vi "PV Curtail Hz.vi"(5 "1/I":dbl=1.0, 6 "PVCurtailEnable":bool, 7 "P":dbl=0.01, 8 "Error In":errorcluster, 9 "reinitialize? (F)":bool, 10 "Current Limit Output":T2, 11 "FPGA Data":T1 {"SSG Active Current" format="%2.1f"; "PV Reactive Power (L1)" format="%2.1f"; "PV Reactive Power (L2)" format="%2.1f"; "PV Total Reactive Power" format="%2.1f"; "Gen Reactive Power (L1)" format="%2.1f"; "Gen Reactive Power (L2)" format="%2.1f"; "Gen Total Reactive Power" format="%2.1f"; "SSG Reactive Power (L1)" format="%2.1f"; "SSG Reactive Power (L2)" format="%2.1f"; "SSG Total Reactive Power" format="%2.1f"; "PV Total Current" format="%2.1f"; "PV Total Voltage" format="%2.1f"; "PV Active Power (L1)" format="%2.1f"; "PV Active Power (L2)" format="%2.1f"; "PV App Power (L1)" format="%2.1f"; "PV App Power (L2)" format="%2.1f"; "PV Total Active Power" format="%2.1f"; "PV Total App Power" format="%2.1f"; "PV Arms (L1)" format="%2.1f"; "PV Arms (L2)" format="%2.1f"; "PV Vrms (L1)" format="%2.1f"; "PV Vrms (L2)" format="%2.1f"; "Gen Total Current" format="%2.1f"; "SSG Total Current" format="%2.1f"; "Gen Total Voltage" format="%2.1f"; "SSG Total Voltage" format="%2.1f"; "Gen Active Power (L1)" format="%2.1f"; "Gen Active Power (L2)" format="%2.1f"; "SSG Active Power (L1)" format="%2.1f"; "SSG Active Power (L2)" format="%2.1f"; "Gen App Power (L1)" format="%2.1f"; "Gen App Power (L2)" format="%2.1f"; "SSG App Power (L1)" format="%2.1f"; "SSG App Power (L2)" format="%2.1f"; "Gen Total Active Power" format="%2.1f"; "Gen Total App Power" format="%2.1f"; "Gen Arms (L1)" format="%2.1f"; "Gen Arms (L2)" format="%2.1f"; "Gen Vrms (L1)" format="%2.1f"; "Gen Vrms (L2)" format="%2.1f"; "SSG Total Active Power" format="%2.1f"; "SSG Total App Power" format="%2.1f"; "SSG Arms (L1)" format="%2.1f"; "SSG Arms (L2)" format="%2.1f"; "SSG Vrms (L1)" format="%2.1f"; "SSG Vrms (L2)" format="%2.1f"}) -> (0 "Error Out":errorcluster, 3 "Frequency Setpoint":sgl)   [LabVIEW 2014]
uses:
  Controls/Current Limit Output.ctl
  Controls/FPGA Data.ctl
  <vilib>/functionblocks/Control/PID/PID.vi
  <vilib>/functionblocks/FB Core/FB Core.xnode
  <vilib>/functionblocks/NI_FunctionBlock Libraries.lvlib
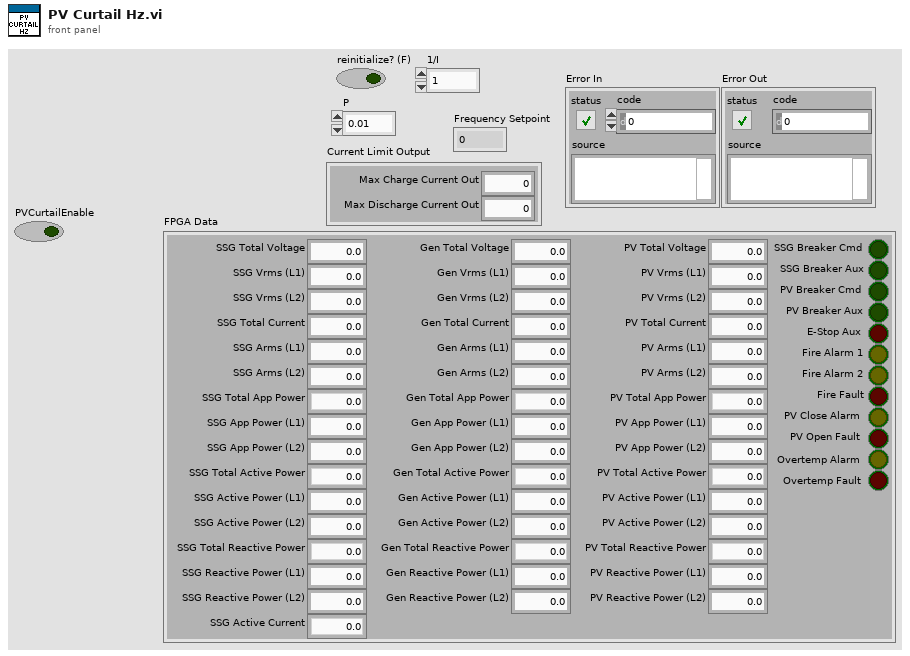
[diagram p1: front panel]
types:
  T1 = typedef "FPGA Data.ctl" = cluster{"Gen Total Voltage":dbl, "Gen Vrms (L1)":dbl, "Gen Vrms (L2)":dbl, "Gen Total Current":dbl, "Gen Arms (L1)":dbl, "Gen Arms (L2)":dbl, "Gen Total App Power":dbl, "Gen App Power (L1)":dbl, "Gen App Power (L2)":dbl, "Gen Total Active Power":dbl, "Gen Active Power (L1)":dbl, "Gen Active Power (L2)":dbl, "Gen Total Reactive Power":dbl, "Gen Reactive Power (L1)":dbl, "Gen Reactive Power (L2)":dbl, "SSG Total Voltage":dbl, "SSG Vrms (L1)":dbl, "SSG Vrms (L2)":dbl, "SSG Total Current":dbl, "SSG Arms (L1)":dbl, "SSG Arms (L2)":dbl, "SSG Total App Power":dbl, "SSG App Power (L1)":dbl, "SSG App Power (L2)":dbl, "SSG Total Active Power":dbl, "SSG Active Power (L1)":dbl, "SSG Active Power (L2)":dbl, "SSG Total Reactive Power":dbl, "SSG Reactive Power (L1)":dbl, "SSG Reactive Power (L2)":dbl, "PV Total Voltage":dbl, "PV Vrms (L1)":dbl, "PV Vrms (L2)":dbl, "PV Total Current":dbl, "PV Arms (L1)":dbl, "PV Arms (L2)":dbl, "PV Total App Power":dbl, "PV App Power (L1)":dbl, "PV App Power (L2)":dbl, "PV Total Active Power":dbl, "PV Active Power (L1)":dbl, "PV Active Power (L2)":dbl, "PV Total Reactive Power":dbl, "PV Reactive Power (L1)":dbl, "PV Reactive Power (L2)":dbl, "SSG Breaker Cmd":bool, "SSG Breaker Aux":bool, "PV Breaker Cmd":bool, "PV Breaker Aux":bool, "E-Stop Aux":bool, "Fire Alarm 1":bool, "Fire Alarm 2":bool, "Fire Fault":bool, "PV Close Alarm":bool, "SSG Active Current":dbl, "Overtemp Alarm":bool, "Overtemp Fault":bool, "PV Open Fault":bool}
  T2 = typedef "Current Limit Output.ctl" = cluster{"Max Charge Current Out":dbl, "Max Discharge Current Out":dbl}
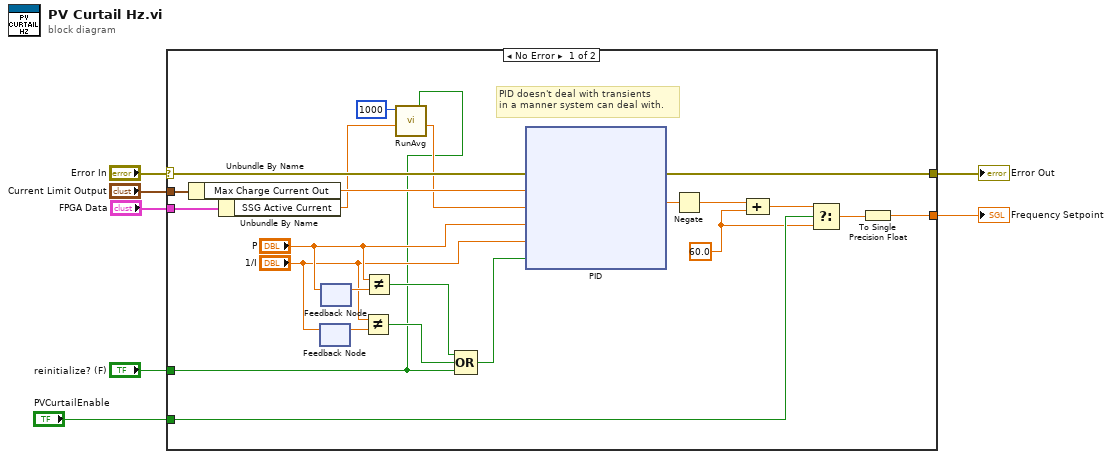
[diagram p0: block diagram]
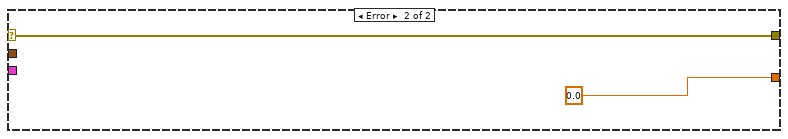
[diagram p2: hidden frame]
diagram:
  n1 = case shown="No Error" "Error In" {
    selector: "Error In" -> [w30 w98]
    tunnel: [w29 w98] -> w6
    tunnel: "Current Limit Output" -> [w28 _]
    tunnel: [w26 sgl 0.0 ("Frequency Setpoint")] -> w4
    tunnel: "reinitialize? (F)" -> [w8 _]
    tunnel: "FPGA Data" -> [w24 _]
    tunnel: "PVCurtailEnable" -> [w14 _]
    frame No Error {
      w13 = 60.0 ("value")
      # "PID doesn't deal with transients\nin a manner system can deal with."
      n2 = Unbundle By Name(w28) -> ("Max Charge Current Out"=w12:dbl)
      n3 = Unbundle By Name(w24) -> ("SSG Active Current"=w10:dbl)
      n4 = feedback #1() -> (w21:dbl)  [unwired: 1 in]
      n5 = feedback-in #1("1/I") -> ()
      n6 = feedback-in #2("P") -> ()
      n7 = feedback #2() -> (w22:dbl)  [unwired: 1 in]
      n8 = Not Equal?(x="1/I", y=w21) -> (x != y?=w19:bool)
      n9 = Not Equal?(x="P", y=w22) -> (x != y?=w18:bool)
      n10 = call "RunAvg.vi"("Ignore avg?"=w8, "value in"=w10, "# of samples"=1000) -> ("value out"=w9:dbl)  [unwired: 4 in]
      n11 = Compound Arithmetic op=OR(w18, w19, w8) -> (w17:bool)
      n12 = xnode "PID"("error in"=w30, "process variable"=w12, "setpoint"=w9, "proportional gain (Kc)"="P", "integral time (Ti, min)"="1/I", "reinitialize? (F)"=w17) -> ("error out"=w29:errorcluster, "output"=w27:dbl)
      n13 = Negate(x=w27) -> (-x=w25:dbl)
      n14 = Compound Arithmetic op=ADD(w25, w13) -> (w16:dbl)
      n15 = Select(t=w16, s=w14, f=w13) -> (s? t:f=w15:dbl)
      n16 = To Single Precision Float(number=w15) -> (single precision float=w26:sgl)
    }
    frame Error {
    }
  }
  "Frequency Setpoint" <- w4
  "Error Out" <- w6
